vi "ROI.vi"(0 "Camera Handle":u32, 1 "Y Start":u32, 2 "Y End":u32, 3 "Y Bin":u32, 11 "error in":errorcluster, 12 "X Start":u32, 13 "X End":u32, 14 "X Bin":u32) -> (4 "Camera Handle":u32, 6 "INI Flag":bool, 10 "String":string, 15 "error out":errorcluster)   [LabVIEW 2015]
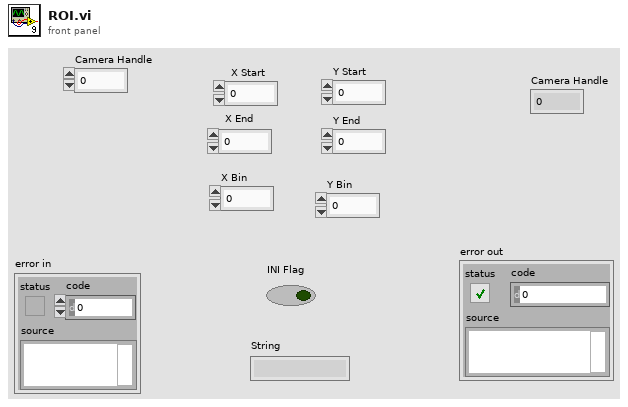
[diagram p1: front panel]
types:
  T1 = cluster{"X Start":u32, "X End":u32, "X Bin":u32, "Y Start":u32, "Y End":u32, "Y Bin":u32}
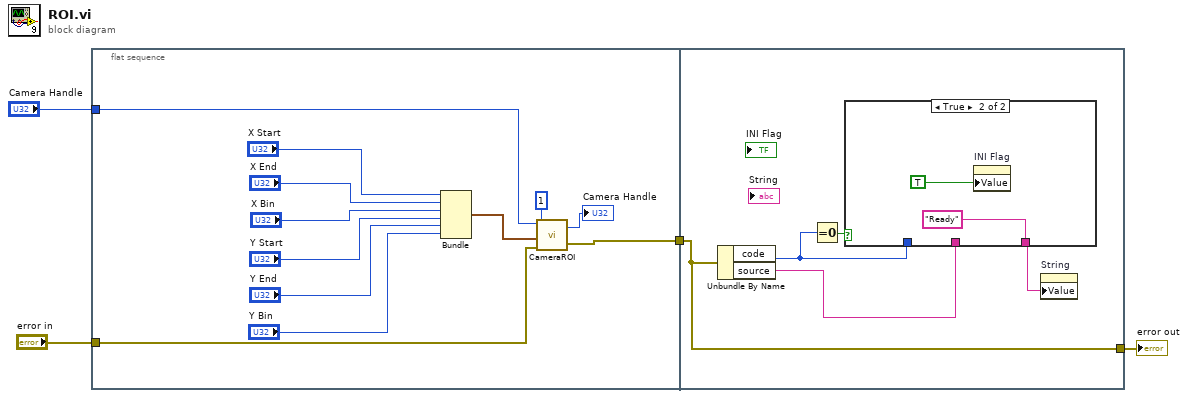
[diagram p0: block diagram]
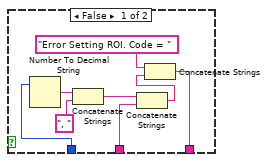
[diagram p2: hidden frame]
diagram:
  n1 = flat-sequence {
    tunnel: "Camera Handle" -> [w13]
    tunnel: [w14] -> w3
    tunnel: "error in" -> [w5]
    tunnel: w3 -> [w18]
    tunnel: [w18] -> w1
    frame #0 {
      n2 = Bundle("X Start"="X Start", "X End"="X End", "X Bin"="X Bin", "Y Start"="Y Start", "Y End"="Y End", "Y Bin"="Y Bin") -> (w16:T1)  [unwired: 1 in]
      n3 = call <userlib>:"CameraROI.vi"("error in"=w5, "ROI Params"=w16, "ROI Index"=1, "Camera Handle"=w13) -> ("error out"=w14:errorcluster, "Camera Handle"=→"Camera Handle":u32)
    }
    frame #1 {
      n4 = Unbundle By Name(w18) -> ("code"=w19:i32, "source"=w20:string)
      n5 = Equal To 0?(x=w19) -> (x = 0?=w21:bool)
      n6 = case shown="True" w21 {
        tunnel: [w22 "Ready"] -> w17
        tunnel: w20 -> [w23 _]
        tunnel: w19 -> [w28 _]
        frame False {
          n7 = Number To Decimal String(number=w28) -> (decimal integer string=w27:string)  [unwired: 1 in]
          n8 = Concatenate Strings(w27, ", ") -> (w24:string)
          n9 = Concatenate Strings(w24, w23) -> (w25:string)
          n10 = Concatenate Strings("Error Setting ROI. Code = ", w25) -> (w22:string)
        }
        frame True {
          n11 = property on="INI Flag" class="Bool (strict)"("Value"=TRUE) -> ()  [unwired: 2 in, 2 out]
        }
      }
      n12 = property on="String" class="Str"("Value"=w17) -> ()  [unwired: 2 in, 2 out]
    }
  }
  "error out" <- w1
